vi "sm.errors.vi"() -> ()   [LabVIEW 2019]
uses:
  <vilib>/rvi/Emulation/niFpgaSctlEmulationGetInTimedLoop.vi
  <vilib>/rvi/Emulation/niFpgaEmulationIsFPGAContextNoSignature.vi
  <vilib>/rvi/DataTransferAndStorage/Container/Common/niFpgaContainerGetUniqueNameForEmu.vi
  <vilib>/rvi/Memory/Memory_Emulation/niFpgaMemoryEmulationCacheClearOnFirstRun.vi
  <vilib>/rvi/Memory/Memory_Emulation/nirvimemoryEmulationManagerCache_MakeExclusive.vi
  <vilib>/rvi/Memory/Memory_Emulation/niFpgaMemoryEmulationValidateCache.vi
  <vilib>/rvi/Memory/Memory_Emulation/nirvimemoryEmulationManagerCache_InsertValue.vi
  <vilib>/Utility/error.llb/Clear Errors.vi
  <vilib>/rvi/Memory/Memory_Emulation/nirvimemoryEmulationManagerCache_ReleaseExclusive.vi
  <vilib>/rvi/Memory/Memory_Emulation/nirvimemoryEmulationManagerCache_GetValue.vi
  <vilib>/rvi/Memory/Memory_Emulation/nirvimemoryEmulationManagerCache_SetValue.vi
  <vilib>/rvi/Emulation/niFpgaProcessEmulError.vi
  rti.global.vi
  <vilib>/rvi/DataTransferAndStorage/Container/XNode/niFpgaContainer.xnode
  <vilib>/rvi/DataTransferAndStorage/Register/Emulation/niFpgaRegisterEmulation.vi
panel:
  out "sub-mode":u8
  out "mode":u8
  out "clear?":bool
  out "mode request":u8
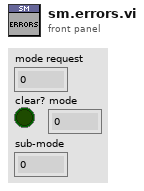
[diagram p1: front panel]
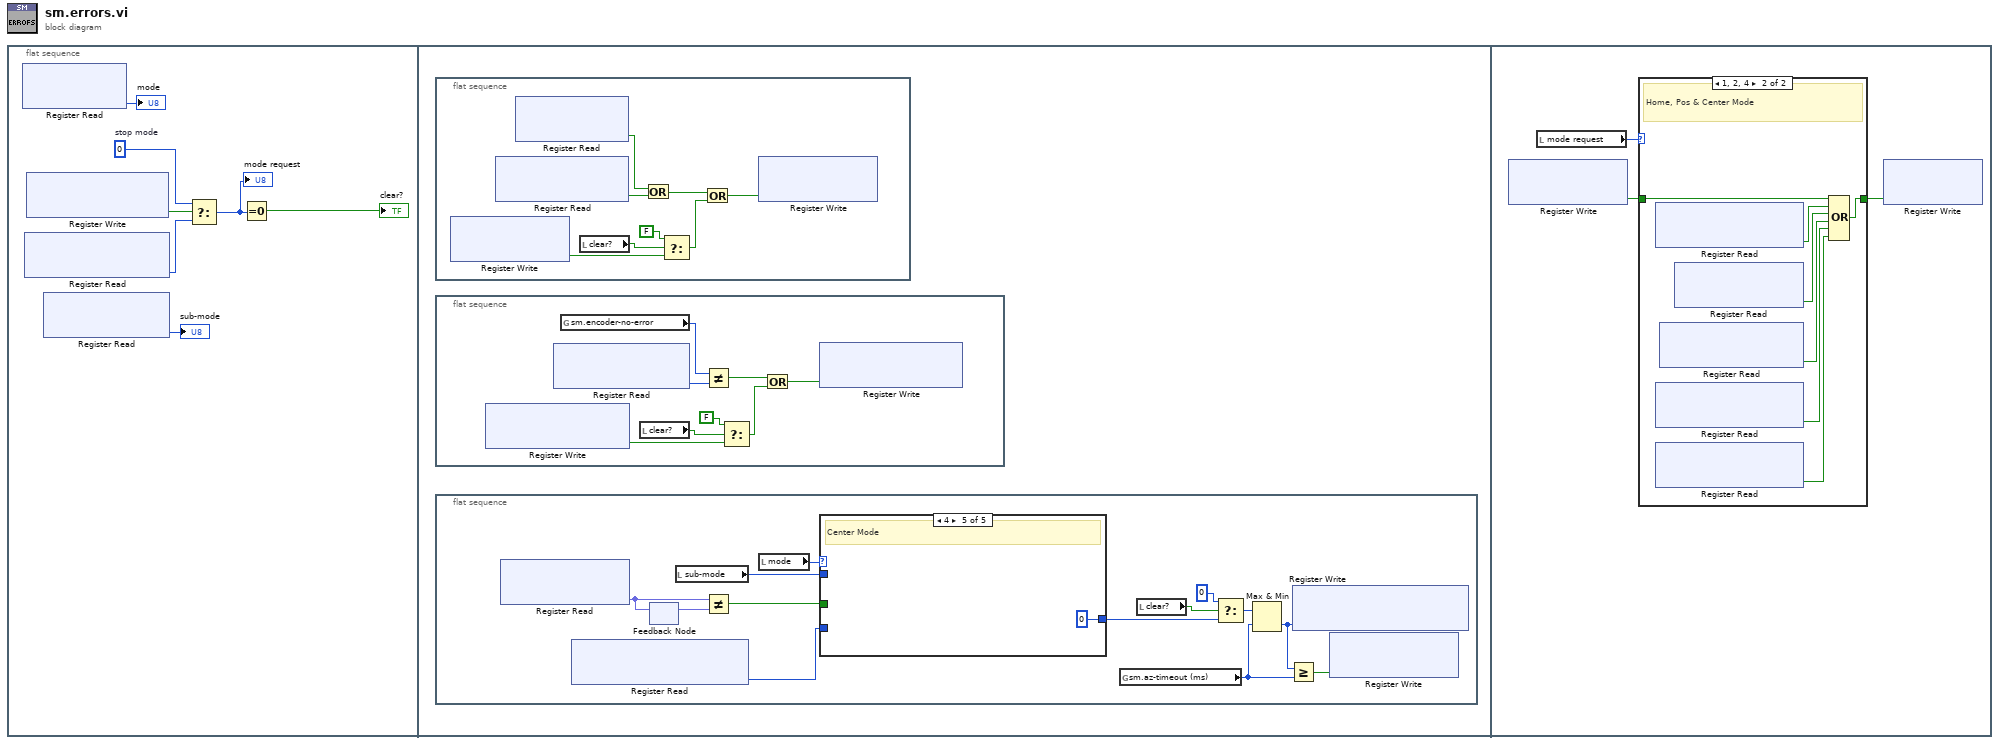
[diagram p0: block diagram]
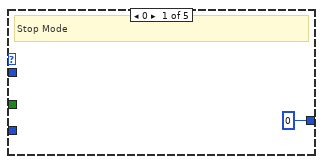
[diagram p2: hidden frame]
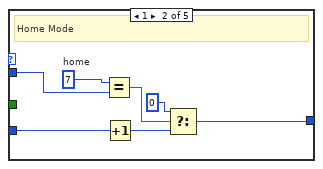
[diagram p3: hidden frame]
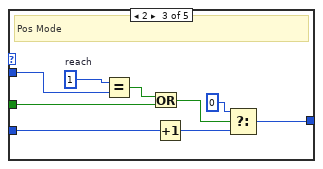
[diagram p4: hidden frame]
diagram:
  n1 = flat-sequence {
    frame #0 {
      w2 = u8 0  # stop mode
      n2 = xnode "Register Read"() -> ("Data"=→"mode":u8)  [unwired: 1 in, 1 out]
      n3 = xnode "Register Read"() -> ("Data"=w3:u8)  [unwired: 1 in, 1 out]
      n4 = xnode "Register Write"() -> ("Data"=w4:bool)  [unwired: 1 in, 1 out]
      n5 = xnode "Register Read"() -> ("Data"=→"sub-mode":u8)  [unwired: 1 in, 1 out]
      n6 = Select(t=w2, s=w4, f=w3) -> (s? t:f=w1:u8)
      "mode request" <- w1
      n7 = Equal To 0?(x=w1) -> (x = 0?=→"clear?":bool)
    }
    frame #1 {
      n8 = flat-sequence {
        frame #0 {
          n9 = xnode "Register Write"() -> ("Data"=w54:bool)  [unwired: 1 in, 1 out]
          n10 = xnode "Register Read"() -> ("Data"=w50:bool)  [unwired: 1 in, 1 out]
          n11 = xnode "Register Read"() -> ("Data"=w49:bool)  [unwired: 1 in, 1 out]
          n12 = local read "clear?"() -> (w55:bool)
          n13 = Or(x=w49, y=w50) -> (x .or. y?=w48:bool)
          n14 = Select(t=FALSE, s=w55, f=w54) -> (s? t:f=w52:bool)
          n15 = Or(x=w48, y=w52) -> (x .or. y?=w51:bool)
          n16 = xnode "Register Write"("Data"=w51) -> ()  [unwired: 1 in, 1 out]
        }
      }
      n17 = flat-sequence {
        frame #0 {
          n18 = xnode "Register Write"() -> ("Data"=w8:bool)  [unwired: 1 in, 1 out]
          n19 = xnode "Register Read"() -> ("Data"=w15:u16)  [unwired: 1 in, 1 out]
          n20 = global read "rti.global.vi" "sm.encoder-no-error"() -> (w14:u16)
          n21 = local read "clear?"() -> (w12:bool)
          n22 = Not Equal?(x=w14, y=w15) -> (x != y?=w11:bool)
          n23 = Select(t=FALSE, s=w12, f=w8) -> (s? t:f=w10:bool)
          n24 = Or(x=w11, y=w10) -> (x .or. y?=w9:bool)
          n25 = xnode "Register Write"("Data"=w9) -> ()  [unwired: 1 in, 1 out]
        }
      }
      n26 = flat-sequence {
        frame #0 {
          n27 = xnode "Register Read"() -> ("Data"=w17:fxp<+/-,32,2>)  [unwired: 1 in, 1 out]
          n28 = xnode "Register Read"() -> ("Data"=w28:u32)  [unwired: 1 in, 1 out]
          n29 = feedback-in #1(w17) -> ()
          n30 = feedback #1() -> (w18:fxp<+/-,32,2>)  [unwired: 1 in]
          n31 = local read "sub-mode"() -> (w19:u8)
          n32 = Not Equal?(x=w17, y=w18) -> (x != y?=w16:bool)
          n33 = local read "mode"() -> (w20:u8)
          n34 = case shown="4" w20 {
            tunnel: w28 -> [_ w31 w42 w46 _]
            tunnel: [u32 0 ("Data") w33 w41 w46 u32 0 ("Data")] -> w23
            tunnel: w19 -> [_ w36 w44 _ _]
            tunnel: w16 -> [_ _ w38 _ _]
            frame 0 {
              # "Stop Mode"
            }
            frame 1 {
              w35 = u8 7  # home
              # "Home Mode"
              n35 = Equal?(x=w35, y=w36) -> (x = y?=w34:bool)
              n36 = Increment(x=w31) -> (x+1=w30:u32)
              n37 = Select(t=u32 0 ("Data"), s=w34, f=w30) -> (s? t:f=w33:u32)
            }
            frame 2 {
              w45 = u8 1  # reach
              # "Pos Mode"
              n38 = Equal?(x=w45, y=w44) -> (x = y?=w39:bool)
              n39 = Or(x=w39, y=w38) -> (x .or. y?=w37:bool)
              n40 = Increment(x=w42) -> (x+1=w43:u32)
              n41 = Select(t=u32 0 ("Data"), s=w37, f=w43) -> (s? t:f=w41:u32)
            }
            frame 3, Default {
              # "Error Mode"
            }
            frame 4 {
              # "Center Mode"
            }
          }
          n42 = global read "rti.global.vi" "sm.az-timeout (ms)"() -> (w26:u32)
          n43 = local read "clear?"() -> (w24:bool)
          n44 = Select(t=u32 0, s=w24, f=w23) -> (s? t:f=w21:u32)
          n45 = Max & Min(x=w21, y=w26) -> (min(x,y)=w27:u32)  [unwired: 1 out]
          n46 = Greater Or Equal?(x=w27, y=w26) -> (x >= y?=w25:bool)
          n47 = xnode "Register Write"("Data"=w27) -> ()  [unwired: 1 in, 1 out]
          n48 = xnode "Register Write"("Data"=w25) -> ()  [unwired: 1 in, 1 out]
        }
      }
    }
    frame #2 {
      n49 = xnode "Register Write"() -> ("Data"=w56:bool)  [unwired: 1 in, 1 out]
      n50 = local read "mode request"() -> (w58:u8)
      n51 = case shown="1, 2, 4" w58 {
        tunnel: w56 -> [w59 w66]
        tunnel: [w59 w63] -> w57
        frame 0, Default {
          # "Stop Mode\nOnly EM disable buttons"
        }
        frame 1, 2, 4 {
          # "Home, Pos & Center Mode"
          n52 = xnode "Register Read"() -> ("Data"=w65:bool)  [unwired: 1 in, 1 out]
          n53 = xnode "Register Read"() -> ("Data"=w61:bool)  [unwired: 1 in, 1 out]
          n54 = xnode "Register Read"() -> ("Data"=w60:bool)  [unwired: 1 in, 1 out]
          n55 = xnode "Register Read"() -> ("Data"=w62:bool)  [unwired: 1 in, 1 out]
          n56 = xnode "Register Read"() -> ("Data"=w64:bool)  [unwired: 1 in, 1 out]
          n57 = Compound Arithmetic op=OR(w66, w65, w64, w62, w61, w60) -> (w63:bool)
        }
      }
      n58 = xnode "Register Write"("Data"=w57) -> ()  [unwired: 1 in, 1 out]
    }
  }
